vi "CreateNv.vi"(0 "NeedleValve in":refnum<class "NeedleValve.lvclass">, 5 "error in (no error)":errorcluster, 7 "FPGA API":refnum<class "FPGA API.lvclass">, 8 "addres":u16=1, 9 "SV_Publisher":refnum<class "SV_Publisher.lvclass">, 11 "ConfigInterface":refnum<class "ConfigInterface.lvclass">, 12 "Tags":T1, 13 "Logger":refnum<class "Logger.lvclass">) -> (14 "NeedleValve out":refnum<class "NeedleValve.lvclass">, 19 "error out":errorcluster)   [LabVIEW 2019, in "NeedleValve.lvclass"]
uses:
  NeedleValve.lvclass
  FPGA_API_class/FPGA API.lvclass
  D:/GIT H4000/H4000/src/Device_class/Device.lvclass
  ConfigInterface_class/ConfigInterface.lvclass
  SV_Puplisher_class/SV_Publisher.lvclass
  Proccess_class/TAGs.ctl
  Logger_class/Logger.lvclass
  TypeDef/Needle Valve Data.ctl
  modbus engine custom/MB_ENGINE_class/Engine State.ctl
  TypeDef/Needle Valve State.ctl
  modbus engine custom/MB_ENGINE_class/Engine Alarms.ctl
  modbus engine custom/MB_ENGINE_class/Settings.ctl
  modbus engine custom/MB_ENGINE_class/Limits Status.ctl
  NeedleValve.lvclass/NeedleValve.ctl
  TypeDef/bool_setting.ctl
  Device_class/Device.lvclass/Device.ctl
  MessageInterface_class/MessageInterface.lvclass
  Device_class/Device.lvclass
  DA_class/DA.lvclass
  Proccess_class/Proccess.lvclass
  modbus engine custom/MB_ENGINE_class/MB_ENGINE.lvclass
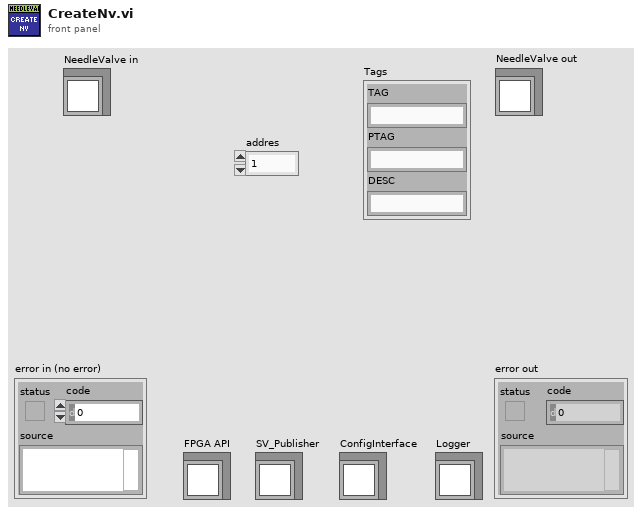
[diagram p1: front panel]
types:
  T1 = typedef "Proccess.lvclass/TAGs.ctl" = cluster{"TAG":string, "PTAG":string, "DESC":string}
  T2 = typedef "bool_setting.ctl" = cluster{"TON_ms":u32, "TOFF_ms":u32}
  T3 = typedef "Needle Valve Data.ctl" = cluster{"Engine State":T4, "StateValveModbus":T5, "Alarms":T6, "RAW":i32, "Angele":dbl, "Step":i32, "Encoder":i32, "Kinematic":T7, "Limits":T8, "EncoderMax":i32, "Counter Max Dont Update":i32, "EncoderMin":i32, "Counter Min Dont Update":i32, "Prepere Counter":i32, "STEP INIT":i32, "offset - Angel":dbl}
  T4 = typedef "MB_ENGINE.lvclass/Engine State.ctl" = u16
  T5 = typedef "Needle Valve State.ctl" = enum16{"STOPED", "CLOSED", "OPENED", "OPENING", "CLOSING", "FULL_CLOSE", "PREP_OPEN"}
  T6 = typedef "MB_ENGINE.lvclass/Engine Alarms.ctl" = cluster{"OL":bool, "TF":bool, "STL":bool, "OCP":bool, "CPUV":bool, "UVLO":bool, "SPI_ERROR":bool, "Fault":bool, "OL 2":bool, "TF 2":bool, "STL 2":bool, "OCP 2":bool, "CPUV 2":bool, "UVLO 2":bool, "reserved":bool, "InitDone":bool}
  T7 = typedef "MB_ENGINE.lvclass/Settings.ctl" = cluster{"ACC Steps Per Sec^2":u16, "DEC Steps Per Sec^2":u16, "Min Velosity Step Per Sec":u16, "Max Velosity Step Per Sec":u16, "MicroStep":u16}
  T8 = typedef "MB_ENGINE.lvclass/Limits Status.ctl" = cluster{"Fault 2 Switch":bool, "Fault 1 Switch":bool, "Center(Home)":bool, "Lower Limit":bool, "Upper Limit":bool}
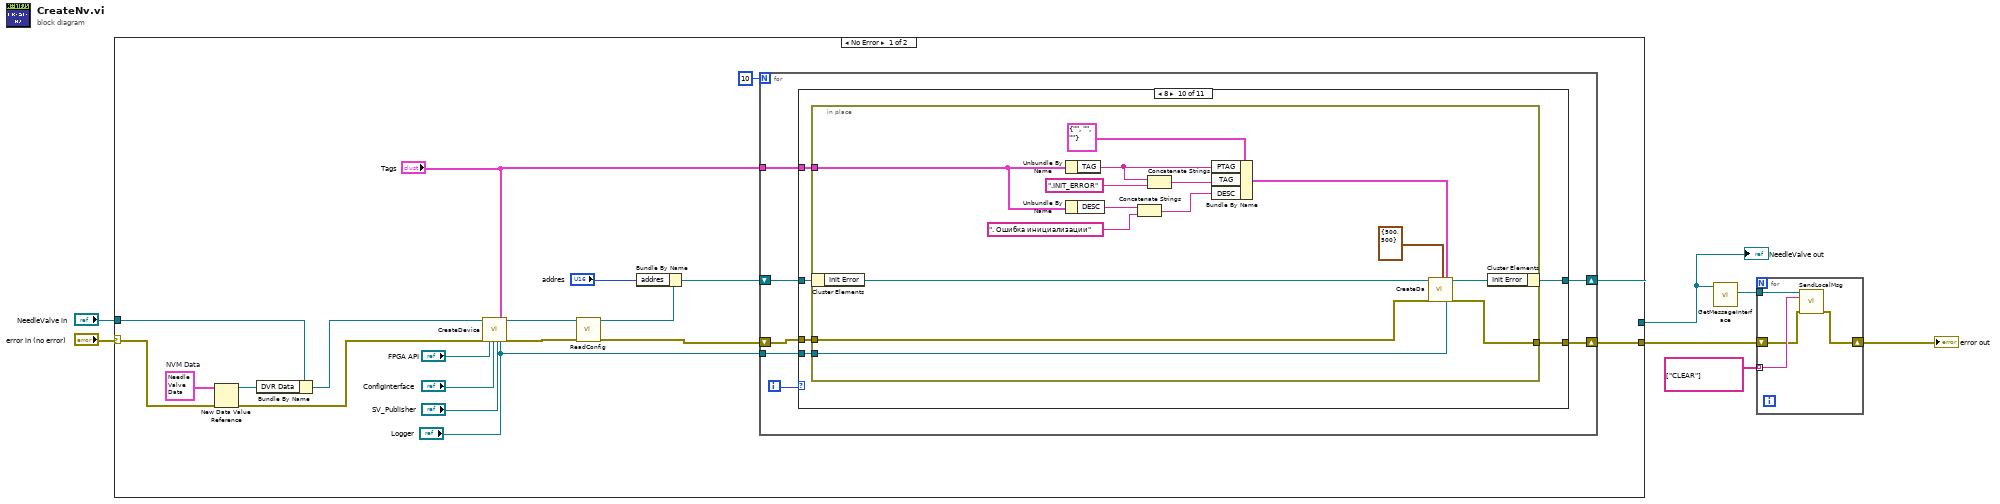
[diagram p0: block diagram]
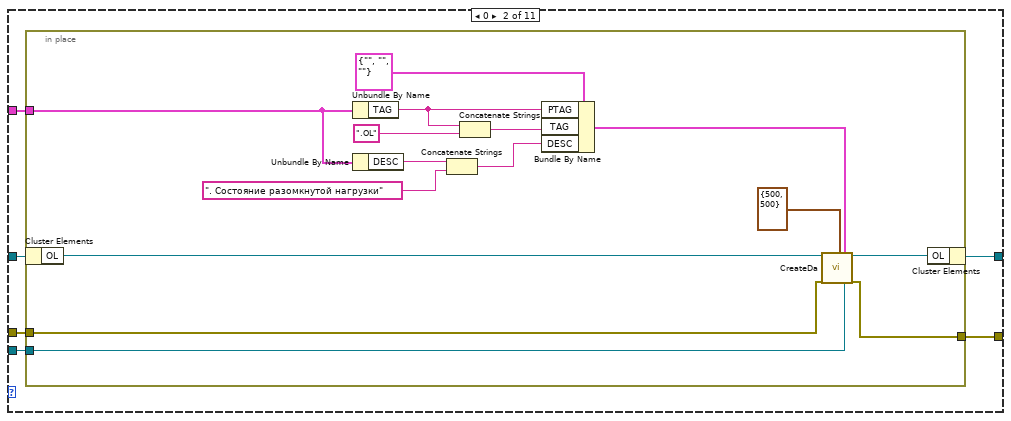
[diagram p3: hidden frame]
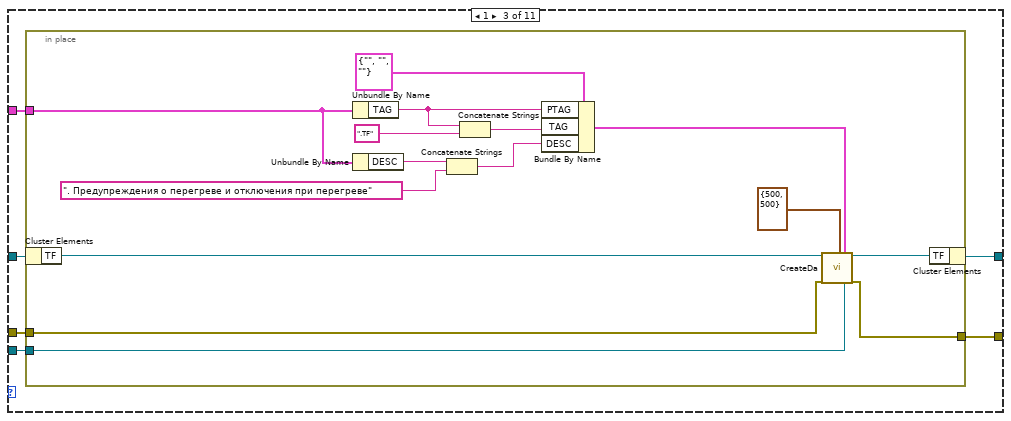
[diagram p4: hidden frame]
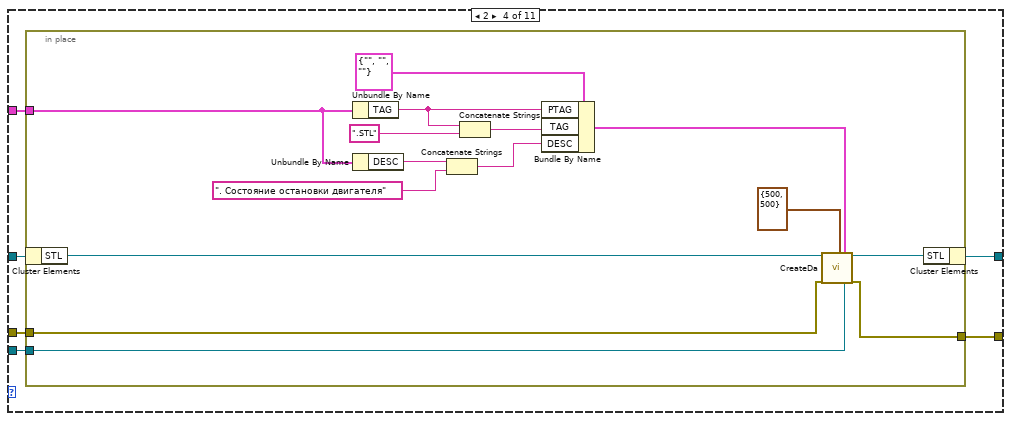
[diagram p5: hidden frame]
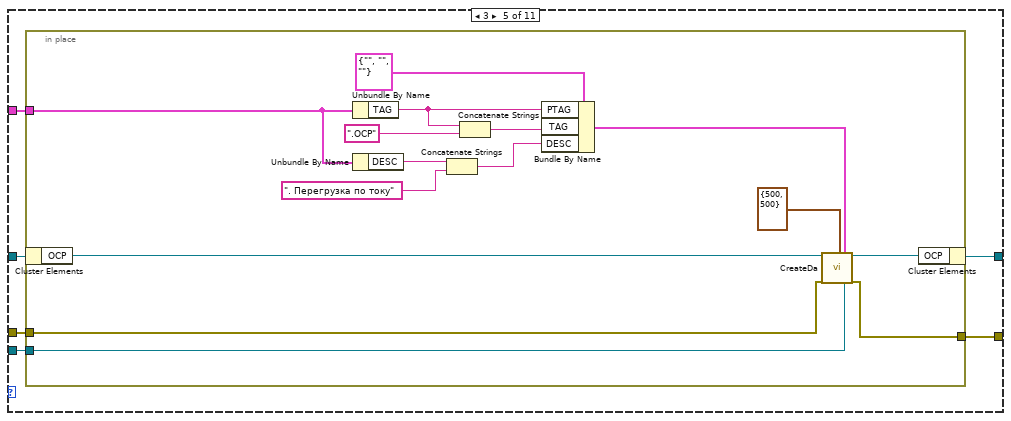
[diagram p6: hidden frame]
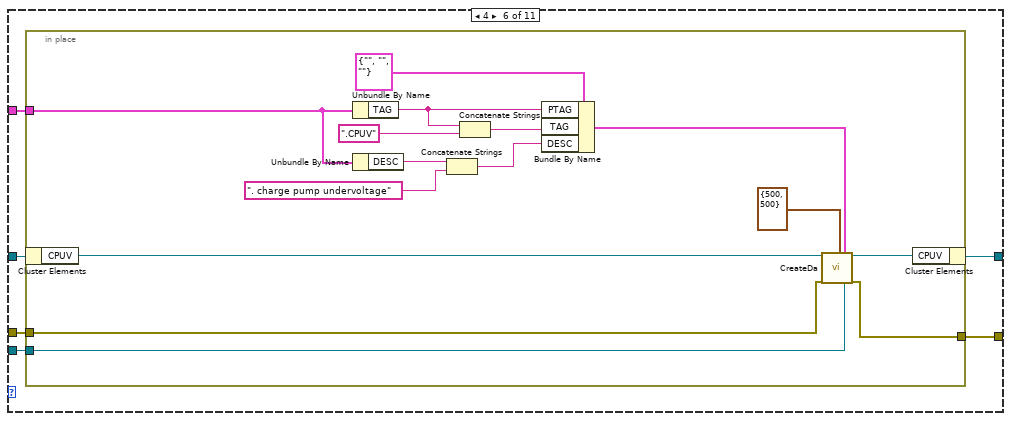
[diagram p7: hidden frame]
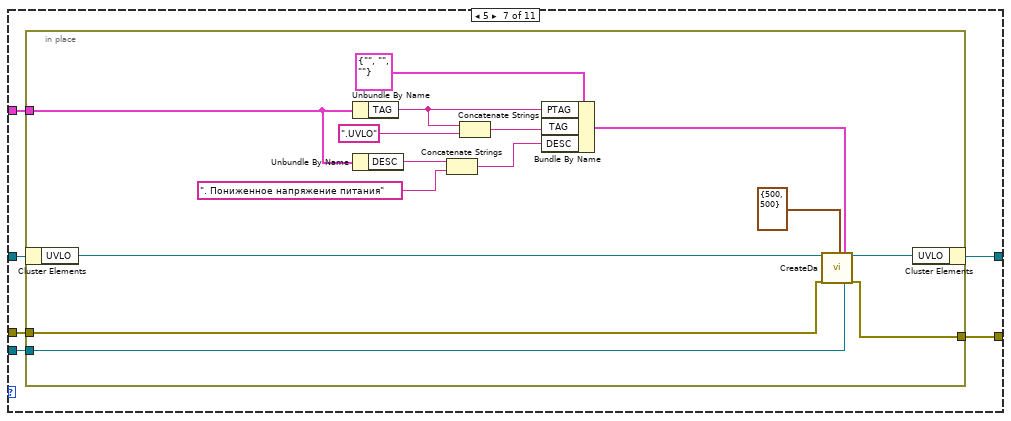
[diagram p8: hidden frame]
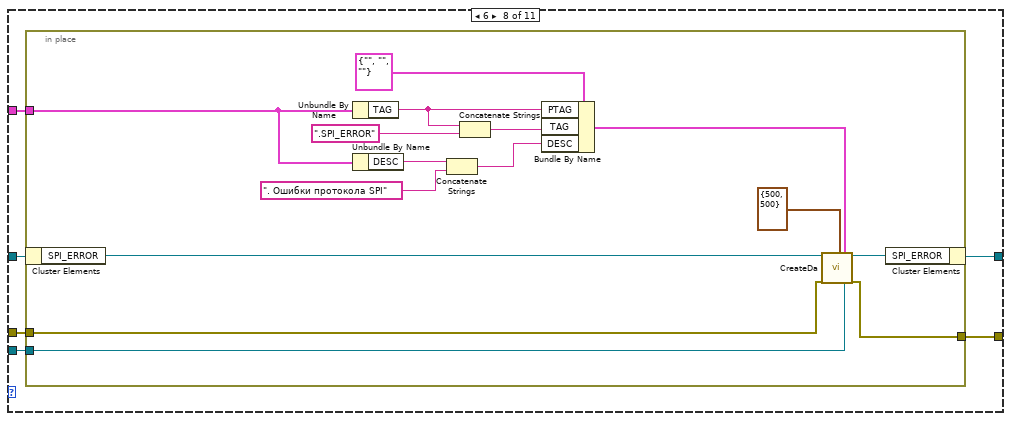
[diagram p9: hidden frame]
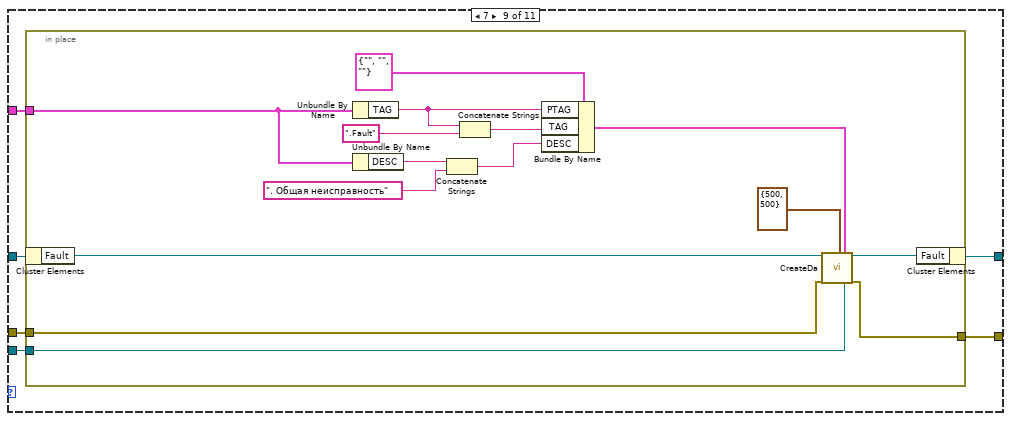
[diagram p10: hidden frame]
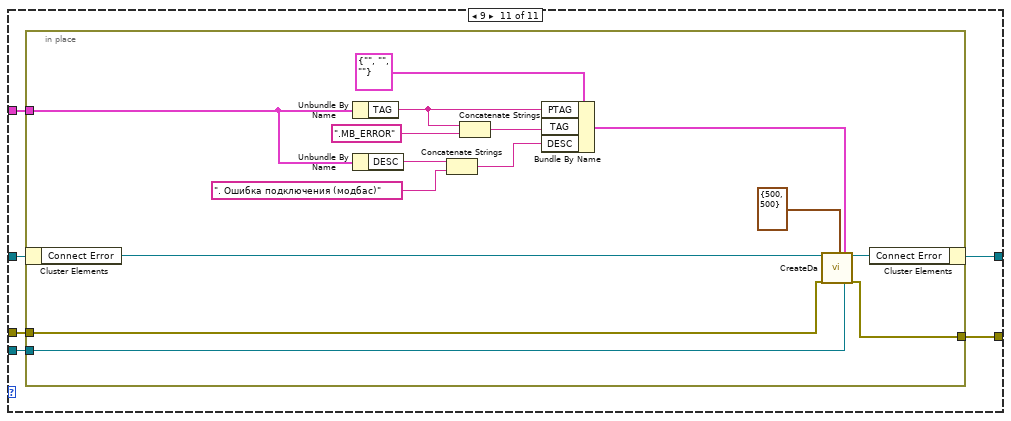
[diagram p11: hidden frame]
diagram:
  n1 = case shown="No Error" "error in (no error)" {
    selector: "error in (no error)" -> [w10 w248]
    tunnel: [w14 w248] -> w3
    tunnel: [w18 w247] -> w1
    tunnel: "NeedleValve in" -> [w26 w247]
    frame No Error {
      w12 = T3 {"Engine State"=8, "StateValveModbus"=enum."STOPED", "Alarms"={"OL"=FALSE, "TF"=FALSE, "STL"=FALSE, "OCP"=FALSE, "CPUV"=FALSE, "UVLO"=FALSE, "SPI_ERROR"=FALSE, "Fault"=FALSE, "OL 2"=FALSE, "TF 2"=FALSE, "STL 2"=FALSE, "OCP 2"=FALSE, "CPUV 2"=FALSE, "UVLO 2"=FALSE, "reserved"=TRUE, "InitDone"=TRUE}, "RAW"=124110, "Angele"=0.0, "Step"=0, "Encoder"=0, "Kinematic"={"ACC Steps Per Sec^2"=100, "DEC Steps Per Sec^2"=100, "Min Velosity Step Per Sec"=100, "Max Velosity Step Per Sec"=200, "MicroStep"=16}, "Limits"={"Fault 2 Switch"=FALSE, "Fault 1 Switch"=FALSE, "Center(Home)"=FALSE, "Lower Limit"=FALSE, "Upper Limit"=FALSE}, "EncoderMax"=0, "Counter Max Dont Update"=0, "EncoderMin"=0, "Counter Min Dont Update"=0, "Prepere Counter"=0, "STEP INIT"=0, "offset - Angel"=0.0}  # NVM Data
      n2 = New Data Value Reference(data value=w12, error in=w10) -> (data value reference=w9:refnum<data-value>, error out=w8:errorcluster)
      n3 = Bundle By Name(cluster=w26, "DVR Data"=w9) -> (w11:refnum<class "NeedleValve.lvclass">)
      n4 = call "CreateDevice.vi"("Device in"=w11, "error in (no error)"=w8, "FPGA API"="FPGA API", "ConfigInterface"="ConfigInterface", "SV_Publisher"="SV_Publisher", "Tags"="Tags", "Logger"="Logger") -> ("Device out"=w25:refnum<class "NeedleValve.lvclass">, "error out"=w24:errorcluster)  [unwired: 11 in]
      n5 = call-dynamic "ReadConfig.vi"("reference in"=w25, "error in (no error)"=w24) -> ("reference out"=w27:refnum<class "NeedleValve.lvclass">, "error out"=w17:errorcluster)  [unwired: 12 in]
      n6 = Bundle By Name(cluster=w27, "addres"="addres") -> (w19:refnum<class "NeedleValve.lvclass">)
      n7 = for {
        N: 10 -> [_]
        tunnel: "Tags" -> [w31]
        tunnel: "Logger" -> [w30]
        shift-right: [w33] -> w18
        shift-left: w19 -> [w34]
        shift-right: [w29] -> w14
        shift-left: w17 -> [w32]
        i -> [w28]
        n8 = case shown="8" w28 {
          tunnel: w34 -> [w36 w42 w63 w84 w105 w126 w147 w168 w189 w210 w231]
          tunnel: [w36 w41 w62 w83 w104 w125 w146 w167 w188 w209 w230] -> w33
          tunnel: w32 -> [w35 w40 w61 w82 w103 w124 w145 w166 w187 w208 w229]
          tunnel: w31 -> [_ w39 w60 w81 w102 w123 w144 w165 w186 w207 w228]
          tunnel: w30 -> [_ w38 w59 w80 w101 w122 w143 w164 w185 w206 w227]
          tunnel: [w35 w37 w58 w79 w100 w121 w142 w163 w184 w205 w226] -> w29
          frame Default {
          }
          frame 0 {
            n9 = in-place {
              in-place-border: w40 -> [w56]
              in-place-border: w39 -> [w46]
              in-place-border: w38 -> [w51]
              in-place-border: [w50] -> w37
              n10 = in-place-cluster #1(w42) -> ("OL"=w57:refnum<class "DA.lvclass">)
              n11 = Unbundle By Name(w46) -> ("TAG"=w49:string)
              n12 = Unbundle By Name(w46) -> ("DESC"=w45:string)
              n13 = Concatenate Strings(w45, ". Состояние разомкнутой нагрузки" ("string")) -> (w43:string)
              n14 = Concatenate Strings(w49, ".OL" ("string")) -> (w47:string)
              n15 = Bundle By Name(cluster=T1 {"TAG"="", "PTAG"="", "DESC"=""} ("Tags"), "PTAG"=w49, "TAG"=w47, "DESC"=w43) -> (w54:T1)
              n16 = call "CreateDa.vi"("Sig_DA in"=w57, "error in (no error)"=w56, "bool_setting"=T2 {"TON_ms"=500, "TOFF_ms"=500}, "Tags"=w54, "Logger"=w51) -> ("Sig_DA out"=w53:refnum<class "DA.lvclass">, "error out"=w50:errorcluster)  [unwired: 13 in]
              n17 = in-place-cluster #1("OL"=w53) -> (w41:refnum<class "NeedleValve.lvclass">)
            }
          }
          frame 1 {
            n18 = in-place {
              in-place-border: w61 -> [w77]
              in-place-border: w60 -> [w67]
              in-place-border: w59 -> [w72]
              in-place-border: [w71] -> w58
              n19 = in-place-cluster #2(w63) -> ("TF"=w78:refnum<class "DA.lvclass">)
              n20 = Unbundle By Name(w67) -> ("TAG"=w70:string)
              n21 = Unbundle By Name(w67) -> ("DESC"=w66:string)
              n22 = Concatenate Strings(w66, ". Предупреждения о перегреве и отключения при перегреве" ("string")) -> (w64:string)
              n23 = Concatenate Strings(w70, ".TF" ("string")) -> (w68:string)
              n24 = Bundle By Name(cluster=T1 {"TAG"="", "PTAG"="", "DESC"=""} ("Tags"), "PTAG"=w70, "TAG"=w68, "DESC"=w64) -> (w75:T1)
              n25 = call "CreateDa.vi"("Sig_DA in"=w78, "error in (no error)"=w77, "bool_setting"=T2 {"TON_ms"=500, "TOFF_ms"=500}, "Tags"=w75, "Logger"=w72) -> ("Sig_DA out"=w74:refnum<class "DA.lvclass">, "error out"=w71:errorcluster)  [unwired: 13 in]
              n26 = in-place-cluster #2("TF"=w74) -> (w62:refnum<class "NeedleValve.lvclass">)
            }
          }
          frame 2 {
            n27 = in-place {
              in-place-border: w82 -> [w98]
              in-place-border: w81 -> [w88]
              in-place-border: w80 -> [w93]
              in-place-border: [w92] -> w79
              n28 = in-place-cluster #3(w84) -> ("STL"=w99:refnum<class "DA.lvclass">)
              n29 = Unbundle By Name(w88) -> ("TAG"=w91:string)
              n30 = Unbundle By Name(w88) -> ("DESC"=w87:string)
              n31 = Concatenate Strings(w87, ". Состояние остановки двигателя" ("string")) -> (w85:string)
              n32 = Concatenate Strings(w91, ".STL" ("string")) -> (w89:string)
              n33 = Bundle By Name(cluster=T1 {"TAG"="", "PTAG"="", "DESC"=""} ("Tags"), "PTAG"=w91, "TAG"=w89, "DESC"=w85) -> (w96:T1)
              n34 = call "CreateDa.vi"("Sig_DA in"=w99, "error in (no error)"=w98, "bool_setting"=T2 {"TON_ms"=500, "TOFF_ms"=500}, "Tags"=w96, "Logger"=w93) -> ("Sig_DA out"=w95:refnum<class "DA.lvclass">, "error out"=w92:errorcluster)  [unwired: 13 in]
              n35 = in-place-cluster #3("STL"=w95) -> (w83:refnum<class "NeedleValve.lvclass">)
            }
          }
          frame 3 {
            n36 = in-place {
              in-place-border: w103 -> [w119]
              in-place-border: w102 -> [w109]
              in-place-border: w101 -> [w114]
              in-place-border: [w113] -> w100
              n37 = in-place-cluster #4(w105) -> ("OCP"=w120:refnum<class "DA.lvclass">)
              n38 = Unbundle By Name(w109) -> ("TAG"=w112:string)
              n39 = Unbundle By Name(w109) -> ("DESC"=w108:string)
              n40 = Concatenate Strings(w108, ". Перегрузка по току" ("string")) -> (w106:string)
              n41 = Concatenate Strings(w112, ".OCP" ("string")) -> (w110:string)
              n42 = Bundle By Name(cluster=T1 {"TAG"="", "PTAG"="", "DESC"=""} ("Tags"), "PTAG"=w112, "TAG"=w110, "DESC"=w106) -> (w117:T1)
              n43 = call "CreateDa.vi"("Sig_DA in"=w120, "error in (no error)"=w119, "bool_setting"=T2 {"TON_ms"=500, "TOFF_ms"=500}, "Tags"=w117, "Logger"=w114) -> ("Sig_DA out"=w116:refnum<class "DA.lvclass">, "error out"=w113:errorcluster)  [unwired: 13 in]
              n44 = in-place-cluster #4("OCP"=w116) -> (w104:refnum<class "NeedleValve.lvclass">)
            }
          }
          frame 4 {
            n45 = in-place {
              in-place-border: w124 -> [w140]
              in-place-border: w123 -> [w130]
              in-place-border: w122 -> [w135]
              in-place-border: [w134] -> w121
              n46 = in-place-cluster #5(w126) -> ("CPUV"=w141:refnum<class "DA.lvclass">)
              n47 = Unbundle By Name(w130) -> ("TAG"=w133:string)
              n48 = Unbundle By Name(w130) -> ("DESC"=w129:string)
              n49 = Concatenate Strings(w129, ". charge pump undervoltage" ("string")) -> (w127:string)
              n50 = Concatenate Strings(w133, ".CPUV" ("string")) -> (w131:string)
              n51 = Bundle By Name(cluster=T1 {"TAG"="", "PTAG"="", "DESC"=""} ("Tags"), "PTAG"=w133, "TAG"=w131, "DESC"=w127) -> (w138:T1)
              n52 = call "CreateDa.vi"("Sig_DA in"=w141, "error in (no error)"=w140, "bool_setting"=T2 {"TON_ms"=500, "TOFF_ms"=500}, "Tags"=w138, "Logger"=w135) -> ("Sig_DA out"=w137:refnum<class "DA.lvclass">, "error out"=w134:errorcluster)  [unwired: 13 in]
              n53 = in-place-cluster #5("CPUV"=w137) -> (w125:refnum<class "NeedleValve.lvclass">)
            }
          }
          frame 5 {
            n54 = in-place {
              in-place-border: w145 -> [w161]
              in-place-border: w144 -> [w151]
              in-place-border: w143 -> [w156]
              in-place-border: [w155] -> w142
              n55 = in-place-cluster #6(w147) -> ("UVLO"=w162:refnum<class "DA.lvclass">)
              n56 = Unbundle By Name(w151) -> ("TAG"=w154:string)
              n57 = Unbundle By Name(w151) -> ("DESC"=w150:string)
              n58 = Concatenate Strings(w150, ". Пониженное напряжение питания" ("string")) -> (w148:string)
              n59 = Concatenate Strings(w154, ".UVLO" ("string")) -> (w152:string)
              n60 = Bundle By Name(cluster=T1 {"TAG"="", "PTAG"="", "DESC"=""} ("Tags"), "PTAG"=w154, "TAG"=w152, "DESC"=w148) -> (w159:T1)
              n61 = call "CreateDa.vi"("Sig_DA in"=w162, "error in (no error)"=w161, "bool_setting"=T2 {"TON_ms"=500, "TOFF_ms"=500}, "Tags"=w159, "Logger"=w156) -> ("Sig_DA out"=w158:refnum<class "DA.lvclass">, "error out"=w155:errorcluster)  [unwired: 13 in]
              n62 = in-place-cluster #6("UVLO"=w158) -> (w146:refnum<class "NeedleValve.lvclass">)
            }
          }
          frame 6 {
            n63 = in-place {
              in-place-border: w166 -> [w182]
              in-place-border: w165 -> [w172]
              in-place-border: w164 -> [w177]
              in-place-border: [w176] -> w163
              n64 = in-place-cluster #7(w168) -> ("SPI_ERROR"=w183:refnum<class "DA.lvclass">)
              n65 = Unbundle By Name(w172) -> ("TAG"=w175:string)
              n66 = Unbundle By Name(w172) -> ("DESC"=w171:string)
              n67 = Concatenate Strings(w171, ". Ошибки протокола SPI" ("string")) -> (w169:string)
              n68 = Concatenate Strings(w175, ".SPI_ERROR" ("string")) -> (w173:string)
              n69 = Bundle By Name(cluster=T1 {"TAG"="", "PTAG"="", "DESC"=""} ("Tags"), "PTAG"=w175, "TAG"=w173, "DESC"=w169) -> (w180:T1)
              n70 = call "CreateDa.vi"("Sig_DA in"=w183, "error in (no error)"=w182, "bool_setting"=T2 {"TON_ms"=500, "TOFF_ms"=500}, "Tags"=w180, "Logger"=w177) -> ("Sig_DA out"=w179:refnum<class "DA.lvclass">, "error out"=w176:errorcluster)  [unwired: 13 in]
              n71 = in-place-cluster #7("SPI_ERROR"=w179) -> (w167:refnum<class "NeedleValve.lvclass">)
            }
          }
          frame 7 {
            n72 = in-place {
              in-place-border: w187 -> [w203]
              in-place-border: w186 -> [w193]
              in-place-border: w185 -> [w198]
              in-place-border: [w197] -> w184
              n73 = in-place-cluster #8(w189) -> ("Fault"=w204:refnum<class "DA.lvclass">)
              n74 = Unbundle By Name(w193) -> ("TAG"=w196:string)
              n75 = Unbundle By Name(w193) -> ("DESC"=w192:string)
              n76 = Concatenate Strings(w192, ". Общая неисправность" ("string")) -> (w190:string)
              n77 = Concatenate Strings(w196, ".Fault" ("string")) -> (w194:string)
              n78 = Bundle By Name(cluster=T1 {"TAG"="", "PTAG"="", "DESC"=""} ("Tags"), "PTAG"=w196, "TAG"=w194, "DESC"=w190) -> (w201:T1)
              n79 = call "CreateDa.vi"("Sig_DA in"=w204, "error in (no error)"=w203, "bool_setting"=T2 {"TON_ms"=500, "TOFF_ms"=500}, "Tags"=w201, "Logger"=w198) -> ("Sig_DA out"=w200:refnum<class "DA.lvclass">, "error out"=w197:errorcluster)  [unwired: 13 in]
              n80 = in-place-cluster #8("Fault"=w200) -> (w188:refnum<class "NeedleValve.lvclass">)
            }
          }
          frame 8 {
            n81 = in-place {
              in-place-border: w208 -> [w224]
              in-place-border: w207 -> [w214]
              in-place-border: w206 -> [w219]
              in-place-border: [w218] -> w205
              n82 = in-place-cluster #9(w210) -> ("Init Error"=w225:refnum<class "DA.lvclass">)
              n83 = Unbundle By Name(w214) -> ("TAG"=w217:string)
              n84 = Unbundle By Name(w214) -> ("DESC"=w213:string)
              n85 = Concatenate Strings(w213, ". Ошибка инициализации" ("string")) -> (w211:string)
              n86 = Concatenate Strings(w217, ".INIT_ERROR" ("string")) -> (w215:string)
              n87 = Bundle By Name(cluster=T1 {"TAG"="", "PTAG"="", "DESC"=""} ("Tags"), "PTAG"=w217, "TAG"=w215, "DESC"=w211) -> (w222:T1)
              n88 = call "CreateDa.vi"("Sig_DA in"=w225, "error in (no error)"=w224, "bool_setting"=T2 {"TON_ms"=500, "TOFF_ms"=500}, "Tags"=w222, "Logger"=w219) -> ("Sig_DA out"=w221:refnum<class "DA.lvclass">, "error out"=w218:errorcluster)  [unwired: 13 in]
              n89 = in-place-cluster #9("Init Error"=w221) -> (w209:refnum<class "NeedleValve.lvclass">)
            }
          }
          frame 9 {
            n90 = in-place {
              in-place-border: w229 -> [w245]
              in-place-border: w228 -> [w235]
              in-place-border: w227 -> [w240]
              in-place-border: [w239] -> w226
              n91 = in-place-cluster #10(w231) -> ("Connect Error"=w246:refnum<class "DA.lvclass">)
              n92 = Unbundle By Name(w235) -> ("TAG"=w238:string)
              n93 = Unbundle By Name(w235) -> ("DESC"=w234:string)
              n94 = Concatenate Strings(w234, ". Ошибка подключения (модбас)" ("string")) -> (w232:string)
              n95 = Concatenate Strings(w238, ".MB_ERROR" ("string")) -> (w236:string)
              n96 = Bundle By Name(cluster=T1 {"TAG"="", "PTAG"="", "DESC"=""} ("Tags"), "PTAG"=w238, "TAG"=w236, "DESC"=w232) -> (w243:T1)
              n97 = call "CreateDa.vi"("Sig_DA in"=w246, "error in (no error)"=w245, "bool_setting"=T2 {"TON_ms"=500, "TOFF_ms"=500}, "Tags"=w243, "Logger"=w240) -> ("Sig_DA out"=w242:refnum<class "DA.lvclass">, "error out"=w239:errorcluster)  [unwired: 13 in]
              n98 = in-place-cluster #10("Connect Error"=w242) -> (w230:refnum<class "NeedleValve.lvclass">)
            }
          }
        }
      }
    }
    frame Error {
    }
  }
  "NeedleValve out" <- w1
  n99 = call "GetMessageInterface.vi"("Device in"=w1) -> ("MessageInterface"=w5:refnum<class "MessageInterface.lvclass">)  [unwired: 10 in]
  n100 = for {
    tunnel: w5 -> [w252]
    tunnel: string[] ["CLEAR"] ("name") -> [w251] mode=indexing
    shift-right: [w249] -> w2
    shift-left: w3 -> [w250]
    n101 = call-dynamic "SendLocalMsg.vi"("reference in"=w252, "name"=w251, "error in (no error)"=w250) -> ("error out"=w249:errorcluster)  [unwired: 10 in, 2 out]
  }
  "error out" <- w2
